vi "Update Cursors from Measurement Cursor Configuration.vi"(11 "State in":T1={"Graph Visible Items"={"Plot Legend"=FALSE, "Scale Legend"=FALSE, "Graph Palette"=FALSE, "Cursor Legend"=FALSE, "X Scrollbar"=FALSE}, "View Table"=FALSE, "Table Visible Items"={"Vertical Scrollbar"=FALSE, "Horizontal Scrollbar"=FALSE, "Row Headers"=FALSE, "Column Headers"=FALSE, "Vertical Lines"=FALSE, "Horizontal Lines"=FALSE}, "Header Font"={"Font Name"="", "Size"=0, "Bold"=FALSE, "Italic"=FALSE, "Underline"=FALSE, "Strikeout"=FALSE, "Color"=0}, "Cell Font"={"Font Name"="", "Size"=0, "Bold"=FALSE, "Italic"=FALSE, "Underline"=FALSE, "Strikeout"=FALSE, "Color"=0}, "Description and Tip..."={"Description"="", "Tip"=""}, "Moveable Splitter Position"=0, "Measurement Cursor Configuration"={"XY"={"enable XY"=FALSE, "Position (X)"=[], "Type"=enum."Absolute", "Y reference"=0.0, "color"=0}, "band"={"enable band"=FALSE, "B1"=0.0, "B2"=0.0, "Fixed bandwidth (B2-B1)"=0.0, "B1 color"=0, "B2 color"=0}, "harmonic"={"enable harmonics"=FALSE, "X reference (1X)"=0.0, "Maximum"=0, "Subset"=enum."All", "1X color"=0, "MX color"=0}, "sideband"={"enable sideband"=FALSE, "X center (C)"=0.0, "Sidebands"=0, "X spacing (s)"=0.0, "Center color"=0, "Sideband color"=0}}, "Cursors"={"List"=[], "Tags"=[]}, "X Increment"=0.0, "X Scale"={"Label Visible"=FALSE, "Label Text"="", "Mapping Mode"=0, "Format String"=""}, "Y Scale"={"Label Visible"=FALSE, "Label Text"="", "Mapping Mode"=0, "Format String"=""}, "Colors"={"background"=16777215, "major grid"=8355711, "minor grid"=12632256, "font"=0}, "desired spectrum view"={"scaling"={"linear/dB"=enum."no change", "dB reference"=0.0, "power/magnitude"=enum."no change", "view"=enum."no change"}, "spectral density"=enum."no change"}, "Plot Color Wheel"=[3381759, 32768, 982784, 4375295, 13827953, 13457919, 16757522, 4343295, 16728758, 12095254], "Plots"=[], "registered user events"=variant, "Lock 1X to Peak"=FALSE, "spectrum component"=32, "phase spectrum view"={"desired units"=0, "desired wrapping"=4}} caption="State" {"phase spectrum view"."desired wrapping" items=["No change", "Unwrap", "Wrap: -360 to 0", "Wrap: -270 to 90", "Wrap: -180 to 180", "Wrap: -90 to 270", "Wrap: 0 to 360", "Wrap: custom range"]; "phase spectrum view"."desired units" items=["No change", "Radians", "Degrees", "Cycles"]; "spectrum component" items=["Magnitude^2"=37, "Magnitude"=32, "Phase"=33, "Real"=34, "Imaginary"=35, "Coherence"=36, "Unknown"=99]; "Y Scale"."Mapping Mode" items=["Linear", "Logarithmic", "dB"]; "X Scale"."Mapping Mode" items=["Linear", "Logarithmic"]}) -> (3 "State out":T1={"Graph Visible Items"={"Plot Legend"=FALSE, "Scale Legend"=FALSE, "Graph Palette"=FALSE, "Cursor Legend"=FALSE, "X Scrollbar"=FALSE}, "View Table"=FALSE, "Table Visible Items"={"Vertical Scrollbar"=FALSE, "Horizontal Scrollbar"=FALSE, "Row Headers"=FALSE, "Column Headers"=FALSE, "Vertical Lines"=FALSE, "Horizontal Lines"=FALSE}, "Header Font"={"Font Name"="", "Size"=0, "Bold"=FALSE, "Italic"=FALSE, "Underline"=FALSE, "Strikeout"=FALSE, "Color"=0}, "Cell Font"={"Font Name"="", "Size"=0, "Bold"=FALSE, "Italic"=FALSE, "Underline"=FALSE, "Strikeout"=FALSE, "Color"=0}, "Description and Tip..."={"Description"="", "Tip"=""}, "Moveable Splitter Position"=0, "Measurement Cursor Configuration"={"XY"={"enable XY"=FALSE, "Position (X)"=[], "Type"=enum."Absolute", "Y reference"=0.0, "color"=0}, "band"={"enable band"=FALSE, "B1"=0.0, "B2"=0.0, "Fixed bandwidth (B2-B1)"=0.0, "B1 color"=0, "B2 color"=0}, "harmonic"={"enable harmonics"=FALSE, "X reference (1X)"=0.0, "Maximum"=0, "Subset"=enum."All", "1X color"=0, "MX color"=0}, "sideband"={"enable sideband"=FALSE, "X center (C)"=0.0, "Sidebands"=0, "X spacing (s)"=0.0, "Center color"=0, "Sideband color"=0}}, "Cursors"={"List"=[], "Tags"=[]}, "X Increment"=0.0, "X Scale"={"Label Visible"=FALSE, "Label Text"="", "Mapping Mode"=0, "Format String"=""}, "Y Scale"={"Label Visible"=FALSE, "Label Text"="", "Mapping Mode"=0, "Format String"=""}, "Colors"={"background"=16777215, "major grid"=8355711, "minor grid"=12632256, "font"=0}, "desired spectrum view"={"scaling"={"linear/dB"=enum."no change", "dB reference"=0.0, "power/magnitude"=enum."no change", "view"=enum."no change"}, "spectral density"=enum."no change"}, "Plot Color Wheel"=[3381759, 32768, 982784, 4375295, 13827953, 13457919, 16757522, 4343295, 16728758, 12095254], "Plots"=[], "registered user events"=variant, "Lock 1X to Peak"=FALSE, "spectrum component"=32, "phase spectrum view"={"desired units"=0, "desired wrapping"=4}} caption="State" {"phase spectrum view"."desired wrapping" items=["No change", "Unwrap", "Wrap: -360 to 0", "Wrap: -270 to 90", "Wrap: -180 to 180", "Wrap: -90 to 270", "Wrap: 0 to 360", "Wrap: custom range"]; "phase spectrum view"."desired units" items=["No change", "Radians", "Degrees", "Cycles"]; "spectrum component" items=["Magnitude^2"=37, "Magnitude"=32, "Phase"=33, "Real"=34, "Imaginary"=35, "Coherence"=36, "Unknown"=99]; "Y Scale"."Mapping Mode" items=["Linear", "Logarithmic", "dB"]; "X Scale"."Mapping Mode" items=["Linear", "Logarithmic"]})   [LabVIEW 2017, in "Spectrum with Cursors.xctl"]
doc: "Set cursor attributes. Set cursor list for graph. Add cursors [{ref,tags}] to display state."
uses:
  <vilib>/addons/_XControls/Spectrum with Cursors/Spectrum with Cursors.xctl
  <vilib>/addons/_XControls/Spectrum with Cursors/Controls/State.ctl
  <vilib>/Utility/miscctls.llb/LVFontTypeDef.ctl
  <vilib>/addons/_XControls/Spectrum with Cursors/Controls/Measurement Cursor Configuration.ctl
  <vilib>/addons/_NISVFA/_Shared subVIs/Controls/NI Spectrum Component.ctl
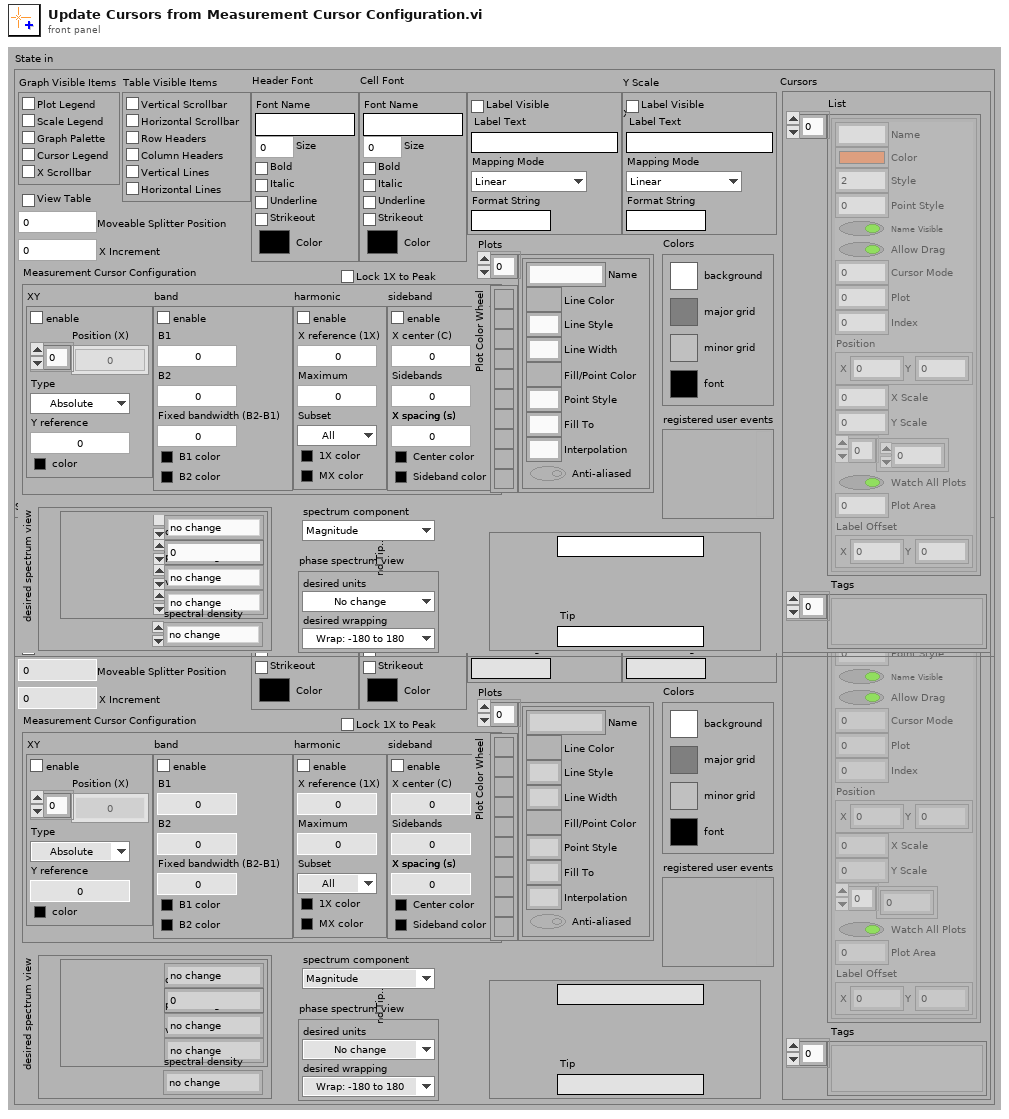
[diagram p1: front panel]
types:
  T1 = typedef "Spectrum with Cursors.xctl/State.ctl" = cluster{"Graph Visible Items":cluster{"Plot Legend":bool, "Scale Legend":bool, "Graph Palette":bool, "Cursor Legend":bool, "X Scrollbar":bool}, "View Table":bool, "Table Visible Items":cluster{"Vertical Scrollbar":bool, "Horizontal Scrollbar":bool, "Row Headers":bool, "Column Headers":bool, "Vertical Lines":bool, "Horizontal Lines":bool}, "Header Font":T2, "Cell Font":T2, "Description and Tip...":cluster{"Description":string, "Tip":string}, "Moveable Splitter Position":i32, "Measurement Cursor Configuration":T3, "Cursors":cluster{"List":cluster{"Name":string, "Color":u32, "Style":i32, "Point Style":u8, "Name Visible":bool, "Allow Drag":bool, "Cursor Mode":u32, "Plot":i32, "Index":i32, "Position":cluster{"X":dbl, "Y":dbl}, "X Scale":u32, "Y Scale":u32, "Watch Plots":i32[], "Watch All Plots":bool, "Plot Area":i32, "Label Offset":cluster{"X":dbl, "Y":dbl}}[], "Tags":variant[]}, "X Increment":dbl, "X Scale":cluster{"Label Visible":bool, "Label Text":string, "Mapping Mode":u8, "Format String":string}, "Y Scale":cluster{"Label Visible":bool, "Label Text":string, "Mapping Mode":u8, "Format String":string}, "Colors":cluster{"background":u32, "major grid":u32, "minor grid":u32, "font":u32}, "desired spectrum view":cluster{"scaling":cluster{"linear/dB":enum16{"no change", "linear", "dB"}, "dB reference":dbl, "power/magnitude":enum16{"no change", "power", "magnitude"}, "view":enum16{"no change", "rms", "peak", "peak-peak"}}, "spectral density":enum16{"no change", "spectrum", "spectral density"}}, "Plot Color Wheel":u32[], "Plots":cluster{"Name":string, "Line Color":u32, "Line Style":u8, "Line Width":u8, "Fill/Point Color":u32, "Point Style":u8, "Fill To":i16, "Interpolation":u8, "Anti-aliased":bool}[], "registered user events":variant, "Lock 1X to Peak":bool, "spectrum component":T4, "phase spectrum view":cluster{"desired units":u16, "desired wrapping":u16}}
  T2 = typedef "LVFontTypeDef.ctl" = cluster{"Font Name":string, "Size":u16, "Bold":bool, "Italic":bool, "Underline":bool, "Strikeout":bool, "Color":u32}
  T3 = typedef "Spectrum with Cursors.xctl/Measurement Cursor Configuration.ctl" = cluster{"XY":cluster{"enable XY":bool, "Position (X)":dbl[], "Type":enum16{"Absolute", "Relative"}, "Y reference":dbl, "color":u32}, "band":cluster{"enable band":bool, "B1":dbl, "B2":dbl, "Fixed bandwidth (B2-B1)":dbl, "B1 color":u32, "B2 color":u32}, "harmonic":cluster{"enable harmonics":bool, "X reference (1X)":dbl, "Maximum":i32, "Subset":enum16{"All", "Even", "Odd"}, "1X color":u32, "MX color":u32}, "sideband":cluster{"enable sideband":bool, "X center (C)":dbl, "Sidebands":i32, "X spacing (s)":dbl, "Center color":u32, "Sideband color":u32}}
  T4 = typedef "NI Spectrum Component.ctl" = u16
  T5 = cluster{"Name":string, "Color":u32, "Style":i32, "Point Style":u8, "Name Visible":bool, "Allow Drag":bool, "Cursor Mode":u32, "Plot":i32, "Index":i32, "Position":cluster{"X":dbl, "Y":dbl}, "X Scale":u32, "Y Scale":u32, "Watch Plots":i32[], "Watch All Plots":bool, "Plot Area":i32, "Label Offset":cluster{"X":dbl, "Y":dbl}}
  T6 = cluster{"Name":string, "Color":u32, "Style":i32, "Point Style":u8, "Name Visible":bool, "Allow Drag":bool, "Cursor Mode":u32, "Plot":i32, "Index":i32, "Position":cluster{"X":dbl, "Y":dbl}, "X Scale":u32, "Y Scale":u32, "Watch Plots":i32[], "Watch All Plots":bool, "Plot Area":i32, "Label Offset":cluster{"X":dbl, "Y":dbl}}[]
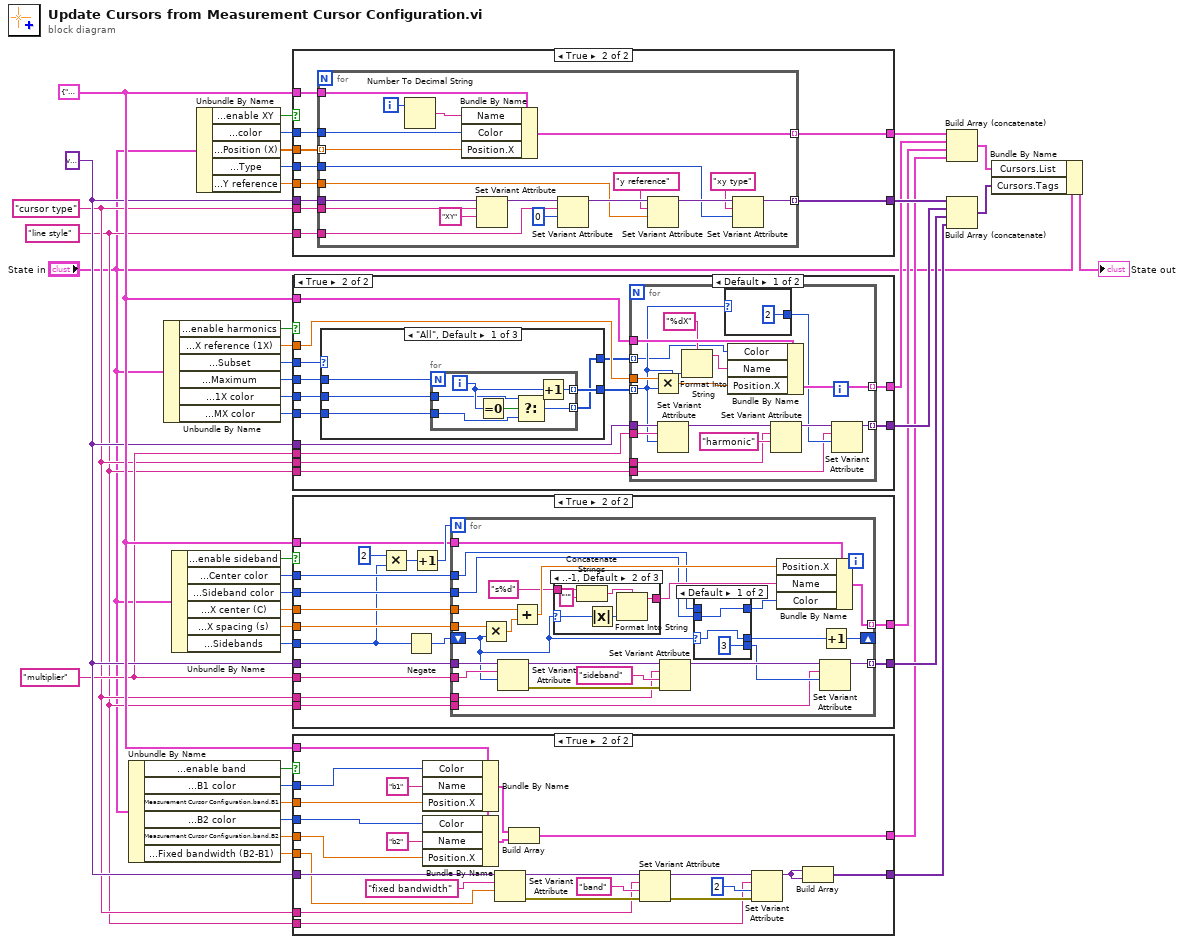
[diagram p0: block diagram]
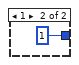
[diagram p4: hidden frame]
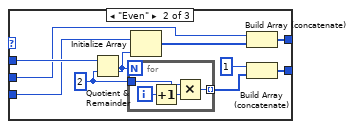
[diagram p5: hidden frame]
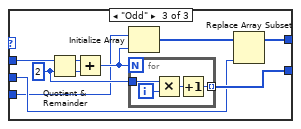
[diagram p6: hidden frame]
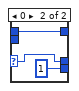
[diagram p8: hidden frame]
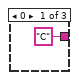
[diagram p9: hidden frame]
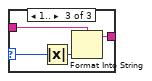
[diagram p10: hidden frame]
diagram:
  w13 = "cursor type"
  w14 = "multiplier"
  w12 = "line style"
  w38 = variant ("tags")
  w39 = T5 {"Name"="", "Color"=16744512, "Style"=2, "Point Style"=0, "Name Visible"=TRUE, "Allow Drag"=TRUE, "Cursor Mode"=0, "Plot"=0, "Index"=0, "Position"={"X"=0.0, "Y"=0.0}, "X Scale"=0, "Y Scale"=0, "Watch Plots"=[], "Watch All Plots"=TRUE, "Plot Area"=0, "Label Offset"={"X"=0.0, "Y"=0.0}}
  n1 = Unbundle By Name("State in") -> ("Measurement Cursor Configuration.band.enable band"=w37:bool, "Measurement Cursor Configuration.band.B1 color"=w33:u32, "Measurement Cursor Configuration.band.B1"=w34:dbl, "Measurement Cursor Configuration.band.B2 color"=w32:u32, "Measurement Cursor Configuration.band.B2"=w36:dbl, "Measurement Cursor Configuration.band.Fixed bandwidth (B2-B1)"=w35:dbl)
  n2 = Unbundle By Name("State in") -> ("Measurement Cursor Configuration.harmonic.enable harmonics"=w25:bool, "Measurement Cursor Configuration.harmonic.X reference (1X)"=w22:dbl, "Measurement Cursor Configuration.harmonic.Subset"=w24:enum16{"All", "Even", "Odd"}, "Measurement Cursor Configuration.harmonic.Maximum"=w23:i32, "Measurement Cursor Configuration.harmonic.1X color"=w20:u32, "Measurement Cursor Configuration.harmonic.MX color"=w21:u32)
  n3 = Unbundle By Name("State in") -> ("Measurement Cursor Configuration.sideband.enable sideband"=w31:bool, "Measurement Cursor Configuration.sideband.Center color"=w27:u32, "Measurement Cursor Configuration.sideband.Sideband color"=w26:u32, "Measurement Cursor Configuration.sideband.X center (C)"=w28:dbl, "Measurement Cursor Configuration.sideband.X spacing (s)"=w30:dbl, "Measurement Cursor Configuration.sideband.Sidebands"=w29:i32)
  n4 = Unbundle By Name("State in") -> ("Measurement Cursor Configuration.XY.enable XY"=w18:bool, "Measurement Cursor Configuration.XY.color"=w15:u32, "Measurement Cursor Configuration.XY.Position (X)"=w19:dbl[], "Measurement Cursor Configuration.XY.Type"=w16:enum16{"Absolute", "Relative"}, "Measurement Cursor Configuration.XY.Y reference"=w17:dbl)
  n5 = case shown="True" w18 {
    tunnel: w39 -> [_ w50]
    tunnel: w19 -> [_ w49]
    tunnel: [_ w48] -> w11
    tunnel: w38 -> [_ w47]
    tunnel: [_ w46] -> w10
    tunnel: w17 -> [_ w45]
    tunnel: w16 -> [_ w44]
    tunnel: w15 -> [_ w43]
    tunnel: w13 -> [_ w42]
    tunnel: w12 -> [_ w41]
    frame False {
    }
    frame True {
      n6 = for {
        tunnel: w50 -> [w60]
        tunnel: w49 -> [w67] mode=indexing
        tunnel: [w69] -> w48 mode=indexing
        tunnel: w47 -> [w65]
        tunnel: [w58] -> w46 mode=indexing
        tunnel: w45 -> [w54]
        tunnel: w44 -> [w56]
        tunnel: w43 -> [w55]
        tunnel: w42 -> [w53]
        tunnel: w41 -> [w52]
        i -> [w68]
        n7 = Number To Decimal String(number=w68) -> (decimal integer string=w51:string)  [unwired: 1 in]
        n8 = Bundle By Name(cluster=w60, "Name"=w51, "Color"=w55, "Position.X"=w67) -> (w69:T5)
        n9 = Set Variant Attribute(Variant=w65, name=w53, value="XY") -> (Variant out=w64:variant)  [unwired: 1 in, 2 out]
        n10 = Set Variant Attribute(Variant=w64, name=w52, value=u8 0 ("Line Style")) -> (Variant out=w62:variant)  [unwired: 1 in, 2 out]
        n11 = Set Variant Attribute(Variant=w62, name="y reference", value=w54) -> (Variant out=w59:variant)  [unwired: 1 in, 2 out]
        n12 = Set Variant Attribute(Variant=w59, name="xy type", value=w56) -> (Variant out=w58:variant)  [unwired: 1 in, 2 out]
      }
    }
  }
  n13 = case shown="True" w25 {
    tunnel: w24 -> [_ w83]
    tunnel: w23 -> [_ w82]
    tunnel: w39 -> [_ w81]
    tunnel: w22 -> [_ w79]
    tunnel: [_ w78] -> w4
    tunnel: w38 -> [_ w77]
    tunnel: [_ w76] -> w9
    tunnel: w14 -> [_ w75]
    tunnel: w21 -> [_ w74]
    tunnel: w20 -> [_ w73]
    tunnel: w13 -> [_ w71]
    tunnel: w12 -> [_ w70]
    frame False {
    }
    frame True {
      n14 = case shown="\"All\", Default" w83 {
        tunnel: w82 -> [w106 w121 w136]
        tunnel: [w107 w122 w137] -> w80
        tunnel: w74 -> [w105 w118 w129]
        tunnel: w73 -> [w104 w115 w131]
        tunnel: [w103 w114 w132] -> w72
        frame "All", Default {
          n15 = for {
            N: w106 -> [_]
            tunnel: [w113] -> w107 mode=indexing
            tunnel: w105 -> [w109]
            tunnel: w104 -> [w110]
            tunnel: [w108] -> w103 mode=indexing
            i -> [w112]
            n16 = Equal To 0?(x=w112) -> (x = 0?=w111:bool)
            n17 = Select(t=w110, s=w111, f=w109) -> (s? t:f=w108:u32)
            n18 = Increment(x=w112) -> (x+1=w113:i32)
          }
        }
        frame "Even" {
          w120 = 2 ("y")
          n19 = Quotient & Remainder(x=w121, y=w120) -> (floor(x/y)=w119:i32)  [unwired: 1 out]
          n20 = for {
            N: w119 -> [_]
            tunnel: [w125] -> w123 mode=indexing
            tunnel: w120 -> [w124]
            i -> [w127]
            n21 = Increment(x=w127) -> (x+1=w126:i32)
            n22 = Multiply(x=w124, y=w126) -> (x*y=w125:i32)
          }
          n23 = Initialize Array(w118, w119) -> (w116:u32[])
          n24 = Build Array (concatenate)(w115, w116) -> (w114:u32[])
          n25 = Build Array (concatenate)(1 ("y"), w123) -> (w122:i32[])
        }
        frame "Odd" {
          w133 = 2 ("y")
          n26 = Quotient & Remainder(x=w136, y=w133) -> (x-y*floor(x/y)=w135:i32, floor(x/y)=w134:i32)
          n27 = Add(x=w135, y=w134) -> (x+y=w130:i32)
          n28 = Initialize Array(w129, w130) -> (w128:u32[])
          n29 = for {
            N: w130 -> [_]
            tunnel: [w139] -> w137 mode=indexing
            tunnel: w133 -> [w138]
            i -> [w141]
            n30 = Multiply(x=w138, y=w141) -> (x*y=w140:i32)
            n31 = Increment(x=w140) -> (x+1=w139:i32)
          }
          n32 = Replace Array Subset(array=w128, new element=w131) -> (w132:u32[])  [unwired: 1 in]
        }
      }
      n33 = for {
        tunnel: w81 -> [w100]
        tunnel: w80 -> [w88] mode=indexing
        tunnel: w79 -> [w99]
        tunnel: [w97] -> w78 mode=indexing
        tunnel: w77 -> [w93]
        tunnel: [w89] -> w76 mode=indexing
        tunnel: w75 -> [w92]
        tunnel: w72 -> [w86] mode=indexing
        tunnel: w71 -> [w85]
        tunnel: w70 -> [w84]
        n34 = Multiply(x=w99, y=w88) -> (x*y=w98:dbl)
        n35 = Set Variant Attribute(Variant=w93, name=w92, value=w88) -> (Variant out=w94:variant)  [unwired: 1 in, 2 out]
        n36 = Format Into String(format string="%dX", w88) -> (resulting string=w96:string)  [unwired: 2 in, 1 out]
        n37 = case shown="Default" w88 {
          tunnel: [u8 2 ("Line Style") u8 1 ("Line Style")] -> w87
          frame Default {
          }
          frame 1 {
          }
        }
        n38 = Bundle By Name(cluster=w100, "Color"=w86, "Name"=w96, "Position.X"=w98) -> (w97:T5)
        n39 = Set Variant Attribute(Variant=w94, name=w85, value="harmonic") -> (Variant out=w90:variant)  [unwired: 1 in, 2 out]
        n40 = Set Variant Attribute(Variant=w90, name=w84, value=w87) -> (Variant out=w89:variant)  [unwired: 1 in, 2 out]
      }
    }
  }
  n41 = case shown="True" w31 {
    tunnel: w30 -> [_ w151]
    tunnel: w29 -> [_ w145]
    tunnel: w39 -> [_ w153]
    tunnel: w28 -> [_ w150]
    tunnel: [_ w152] -> w5
    tunnel: w38 -> [_ w149]
    tunnel: [_ w148] -> w8
    tunnel: w27 -> [_ w147]
    tunnel: w26 -> [_ w146]
    tunnel: w14 -> [_ w144]
    tunnel: w12 -> [_ w143]
    tunnel: w13 -> [_ w142]
    frame False {
    }
    frame True {
      n42 = Multiply(x=2, y=w145) -> (x*y=w156:i32)
      n43 = Negate(x=w145) -> (-x=w154:i32)
      n44 = Increment(x=w156) -> (x+1=w155:i32)
      n45 = for {
        N: w155 -> [_]
        shift-right: [w181] -> _
        shift-left: w154 -> [w166]
        tunnel: w153 -> [w169]
        tunnel: [w179] -> w152 mode=indexing
        tunnel: w151 -> [w178]
        tunnel: w150 -> [w177]
        tunnel: w144 -> [w174]
        tunnel: w149 -> [w173]
        tunnel: [w167] -> w148 mode=indexing
        tunnel: w147 -> [w161]
        tunnel: w146 -> [w160]
        tunnel: w143 -> [w159]
        tunnel: w142 -> [w158]
        n46 = Multiply(x=w178, y=w166) -> (x*y=w176:dbl)
        n47 = Set Variant Attribute(Variant=w173, name=w174, value=w166) -> (Variant out=w170:variant, error out=w171:errorcluster)  [unwired: 1 in, 1 out]
        n48 = Add(x=w177, y=w176) -> (x+y=w175:dbl)
        n49 = case shown="..-1, Default" w166 {
          selector: w166 -> [_ w193 w197]
          tunnel: ["C" w194 w198] -> w180
          tunnel: "s%d" ("format string") -> [_ w191 w195]
          frame 0 {
          }
          frame ..-1, Default {
            n50 = Concatenate Strings(w191, "'" ("string")) -> (w190:string)
            n51 = Absolute Value(x=w193) -> (abs(x)=w192:i32)
            n52 = Format Into String(format string=w190, w192) -> (resulting string=w194:string)  [unwired: 2 in, 1 out]
          }
          frame 1.. {
            n53 = Absolute Value(x=w197) -> (abs(x)=w196:i32)
            n54 = Format Into String(format string=w195, w196) -> (resulting string=w198:string)  [unwired: 2 in, 1 out]
          }
        }
        n55 = Set Variant Attribute(Variant=w170, name=w158, value="sideband", error in=w171) -> (Variant out=w168:variant)  [unwired: 2 out]
        n56 = case shown="Default" w166 {
          selector: w166 -> [w184 w187]
          tunnel: [w184 w187] -> w165
          tunnel: [u8 3 ("Line Style") u8 1 ("Line Style")] -> w164
          tunnel: [w182 w185] -> w162
          tunnel: w161 -> [_ w185]
          tunnel: w160 -> [w182 _]
          frame Default {
          }
          frame 0 {
          }
        }
        n57 = Bundle By Name(cluster=w169, "Position.X"=w175, "Name"=w180, "Color"=w162) -> (w179:T5)
        n58 = Set Variant Attribute(Variant=w168, name=w159, value=w164) -> (Variant out=w167:variant)  [unwired: 1 in, 2 out]
        n59 = Increment(x=w165) -> (x+1=w181:i32)
      }
    }
  }
  n60 = case shown="True" w37 {
    tunnel: w36 -> [_ w218]
    tunnel: w35 -> [_ w212]
    tunnel: w39 -> [_ w207]
    tunnel: w34 -> [_ w219]
    tunnel: [_ w216] -> w6
    tunnel: w38 -> [_ w214]
    tunnel: [_ w211] -> w7
    tunnel: w33 -> [_ w206]
    tunnel: w32 -> [_ w205]
    tunnel: w13 -> [_ w200]
    tunnel: w12 -> [_ w199]
    frame False {
    }
    frame True {
      n61 = Bundle By Name(cluster=w207, "Color"=w206, "Name"="b1" ("format string"), "Position.X"=w219) -> (w215:T5)
      n62 = Bundle By Name(cluster=w207, "Color"=w205, "Name"="b2", "Position.X"=w218) -> (w217:T5)
      n63 = Set Variant Attribute(Variant=w214, name="fixed bandwidth", value=w212) -> (Variant out=w209:variant, error out=w210:errorcluster)  [unwired: 1 in, 1 out]
      n64 = Build Array(w215, w217) -> (w216:T6)
      n65 = Set Variant Attribute(Variant=w209, name=w200, value="band", error in=w210) -> (Variant out=w204:variant, error out=w202:errorcluster)  [unwired: 1 out]
      n66 = Set Variant Attribute(Variant=w204, name=w199, value=u8 2 ("Line Style"), error in=w202) -> (Variant out=w203:variant)  [unwired: 2 out]
      n67 = Build Array(w203, w203) -> (w211:variant[])
    }
  }
  n68 = Build Array (concatenate)(w11, w4, w5, w6) -> (w1:T6)
  n69 = Build Array (concatenate)(w10, w9, w8, w7) -> (w2:variant[])
  n70 = Bundle By Name(cluster="State in", "Cursors.List"=w1, "Cursors.Tags"=w2) -> (→"State out":T1)
